vi "_Get Control Values by Index.vi"(8 "error in (no error)":errorcluster, 10 "control indexes":i32[](array[numeric]), 11 "VI Refnum":refnum<vi>) -> (0 "error out":errorcluster, 9 "data values":variant[](array[variant]))   [LabVIEW 2017, in "TagDB.lvlib"]
uses:
  TagDB.lvlib
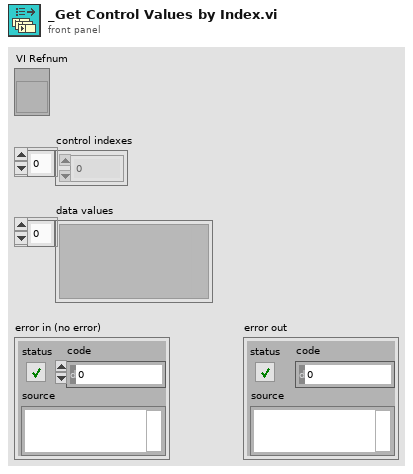
[diagram p1: front panel]
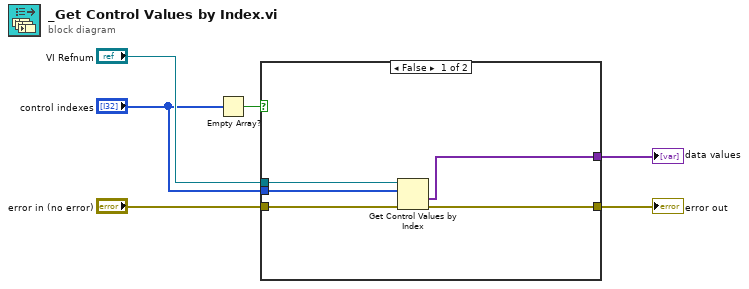
[diagram p0: block diagram]
diagram:
  n1 = Empty Array?(array="control indexes") -> (empty?=w2:bool)
  n2 = case shown="False" w2 {
    tunnel: [w11 w12] -> w6
    tunnel: "error in (no error)" -> [w8 w12]
    tunnel: "VI Refnum" -> [w10 _]
    tunnel: "control indexes" -> [w9 _]
    tunnel: [w7 _] -> w1
    frame False {
      n3 = Get Control Values by Index(0:w10, 1:w9, 3:w8) -> (10:w7:variant[], 11:w11:errorcluster)
    }
    frame True {
    }
  }
  "error out" <- w6
  "data values" <- w1
